vi "PulsedOut.vi"(2 "Cycles":u32=60, 5 "Channel":u16, 6 "frequency (MHz)":dbl=1.367, 7 "error in (no error)":errorcluster, 8 "SEQ IN":u32, 9 "chn num":u16=64, 10 "connection ID":refnum<k5>) -> (0 "error out":errorcluster, 1 "OK?":bool, 3 "connection ID out":refnum<k5>, 4 "SEQ OUT":u32)   [LabVIEW 2016]
panel:
  # "0表示全部打开"
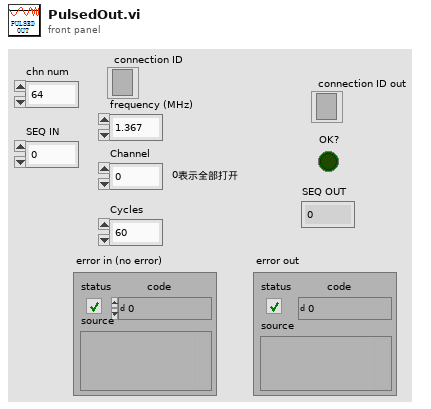
[diagram p1: front panel]
types:
  T1 = enum8{"SET_VOLT", "SET_CHANNEL_VOLT", "SET_PHASE", "START_HEAT", "STOP_HEAT", "CHANNEL_CTRL_SINGLE", "CHANNEL_CTRL_ALL", "READ_VOLT_SET", "READ_VOLT_SET_RSP", "READ_CURRENT_VOLT", "READ_CURRENT_VOLT_RSP", "READ_PHASE", "READ_PHASE_RSP", "READ_HEATTIME_LEFT", "READ_HEATTIME_LEFT_RSP", "EXEC_RSP"}
  T2 = enum8{"SET_VOLT", "SET_CHENNEL_VOLT", "SET_PHASE", "START_HEAT", "STOP_HEAT", "CHANNEL_CTRL_SINGLE", "CHANNEL_CTRL_ALL", "READ_VOLT_SET", "READ_VOLT_SET_RSP", "READ_CURRENT_VOLT", "READ_CURRENT_VOLT_RSP", "READ_PHASE", "READ_PHASE_RSP", "READ_HEATTIME_LEFT", "READ_HEATTIME_LEFT_RSP", "EXEC_RSP"}
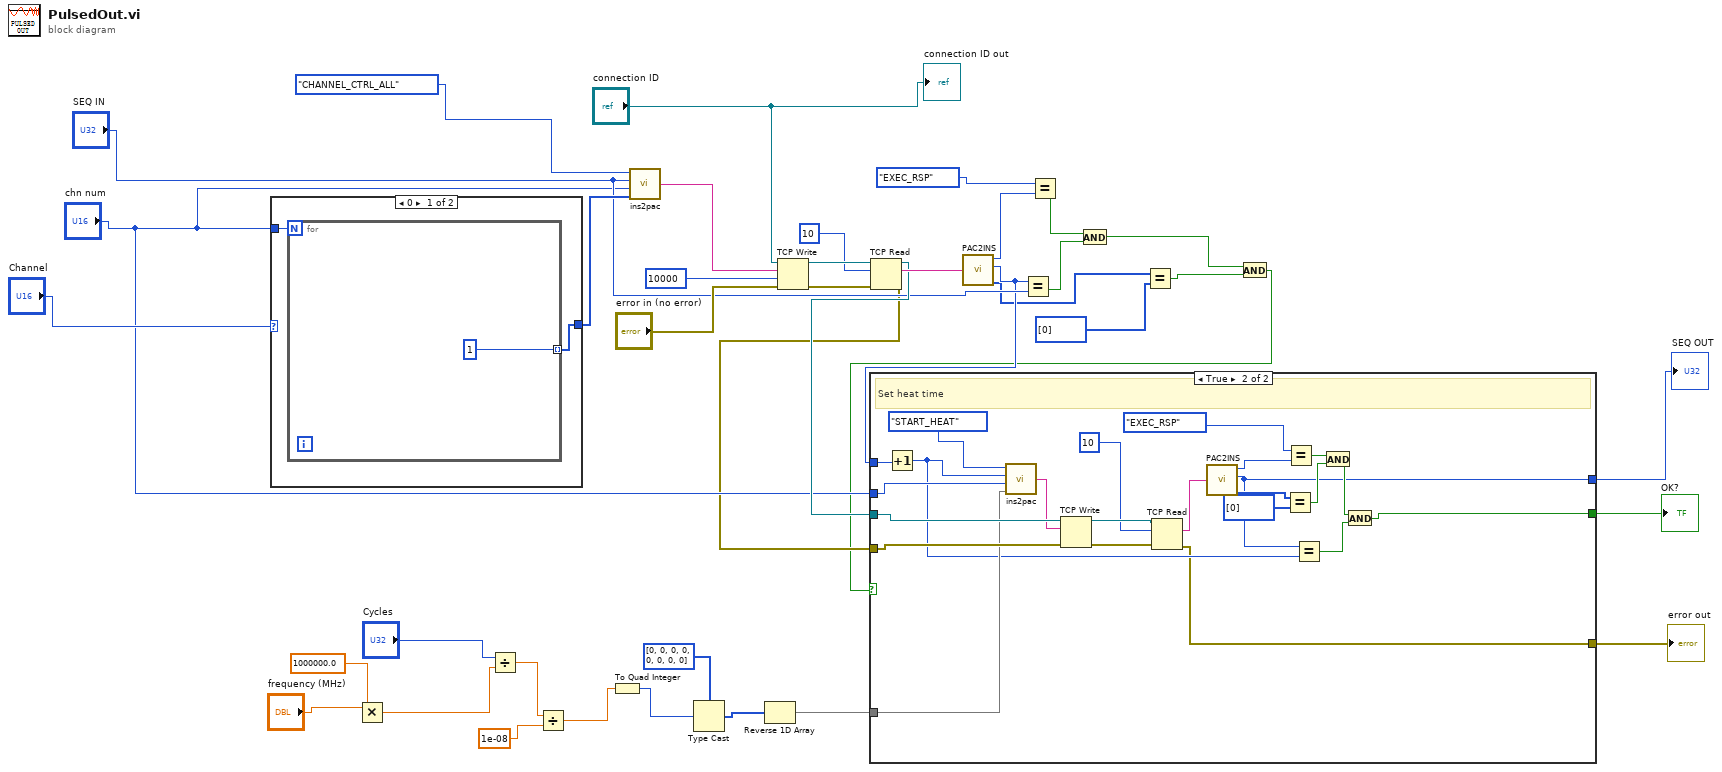
[diagram p0: block diagram]
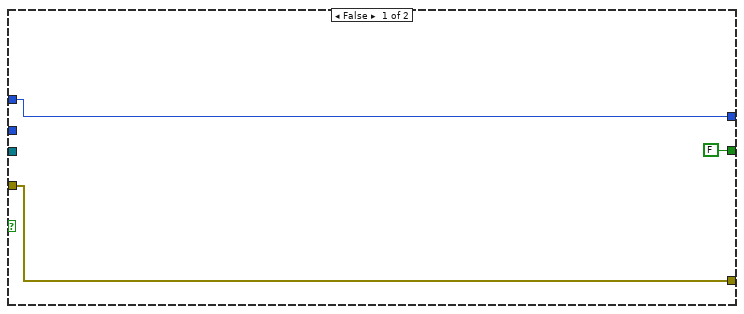
[diagram p2: hidden frame]
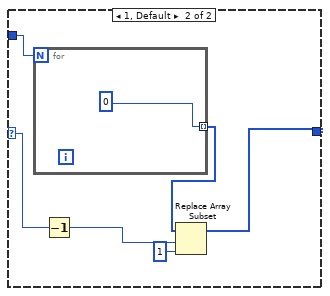
[diagram p3: hidden frame]
diagram:
  n1 = case shown="0" "Channel" {
    selector: "Channel" -> [_ w47]
    tunnel: "chn num" -> [w41 w48]
    tunnel: [w40 w43] -> w38
    frame 0 {
      n2 = for {
        N: w41 -> [_]
        tunnel: [1] -> w40 mode=indexing
      }
    }
    frame 1, Default {
      n3 = for {
        N: w48 -> [_]
        tunnel: [0] -> w46 mode=indexing
      }
      n4 = Decrement(x=w47) -> (x-1=w45:u16)
      n5 = Replace Array Subset(array=w46, new element=1 ("new element/subarray"), index=w45) -> (w43:i32[])
    }
  }
  n6 = Multiply(x="frequency (MHz)", y=1000000.0) -> (x*y=w20:dbl)
  n7 = Divide(x="Cycles", y=w20) -> (x/y=w19:dbl)
  n8 = Divide(x=w19, y=1e-08) -> (x/y=w17:dbl)
  n9 = To Quad Integer(1:w17) -> (0:w15:i64)
  n10 = call "ins2pac.vi"("BODY"=w38, "chn num"="chn num", "SEQUENCE"="SEQ IN", "TYPE"=T1."CHANNEL_CTRL_ALL") -> ("PACKET"=w37:string)
  n11 = Type Cast(type=u8[] [0, 0, 0, 0, 0, 0, 0, 0], x=w15) -> (*(type *) &x=w14:u8[])
  n12 = Reverse 1D Array(array=w14) -> (reversed array=w13:u8[])
  n13 = TCP Write(connection ID="connection ID", data in=w37, error in (no error)="error in (no error)", 9:10000 ("timeout ms (25000)")) -> (connection ID out=w33:refnum<k5>, error out=w34:errorcluster)  [unwired: 1 out]
  n14 = TCP Read(connection ID=w33, bytes to read=10, error in (no error)=w34) -> (connection ID out=w27:refnum<k5>, data out=w31:string, error out=w24:errorcluster)  [unwired: 2 in]
  n15 = call "PAC2INS.vi"("PACKET"=w31) -> ("TYPE"=w30:T2, "SEQUENCE"=w12:u32, "BODY"=w11:u8[])  [unwired: 1 out]
  n16 = Equal?(x=w12, y="SEQ IN") -> (x = y?=w28:bool)
  n17 = Equal?(x=T1."EXEC_RSP" ("TYPE"), y=w30) -> (x = y?=w29:bool)
  n18 = And(x=w29, y=w28) -> (x .and. y?=w10:bool)
  n19 = Equal?(x=w11, y=i32[] [0]) -> (x = y?=w9:bool)
  n20 = And(x=w10, y=w9) -> (x .and. y?=w8:bool)
  n21 = case shown="True" w8 {
    tunnel: w27 -> [_ w75]
    tunnel: w12 -> [w50 w74]
    tunnel: "chn num" -> [_ w73]
    tunnel: w24 -> [w51 w71]
    tunnel: w13 -> [_ w70]
    tunnel: [FALSE w57] -> w6
    tunnel: [w51 w56] -> w5
    tunnel: [w50 w55] -> w3
    frame False {
    }
    frame True {
      # "Set heat time"
      n22 = Increment(x=w74) -> (x+1=w64:u32)
      n23 = call "ins2pac.vi"("BODY"=w70, "chn num"=w73, "SEQUENCE"=w64, "TYPE"=T1."START_HEAT") -> ("PACKET"=w72:string)
      n24 = TCP Write(connection ID=w75, data in=w72, error in (no error)=w71) -> (connection ID out=w69:refnum<k5>, error out=w67:errorcluster)  [unwired: 1 in, 1 out]
      n25 = TCP Read(connection ID=w69, bytes to read=10, error in (no error)=w67) -> (data out=w66:string, error out=w56:errorcluster)  [unwired: 2 in, 1 out]
      n26 = call "PAC2INS.vi"("PACKET"=w66) -> ("TYPE"=w65:T2, "SEQUENCE"=w55:u32, "BODY"=w63:u8[])  [unwired: 1 out]
      n27 = Equal?(x=w63, y=u8[] [0]) -> (x = y?=w60:bool)
      n28 = Equal?(x=T1."EXEC_RSP" ("TYPE"), y=w65) -> (x = y?=w61:bool)
      n29 = Equal?(x=w55, y=w64) -> (x = y?=w58:bool)
      n30 = And(x=w61, y=w60) -> (x .and. y?=w59:bool)
      n31 = And(x=w59, y=w58) -> (x .and. y?=w57:bool)
    }
  }
  "error out" <- w5
  "OK?" <- w6
  "SEQ OUT" <- w3
  "connection ID out" <- "connection ID"
